vi "Upate Power.vi"(8 "error in":errorcluster, 11 "Refnum in":refnum<k21>) -> (0 "error out":errorcluster, 3 "Refnum out":refnum<k21>)   [LabVIEW 2015]
uses:
  <vilib>/DAQmx/write.llb/DAQmx Write (Digital 1D Bool NChan 1Samp 1Line).vi
  <vilib>/DAQmx/miscellaneous.llb/DAQmx Fill In Error Info.vi
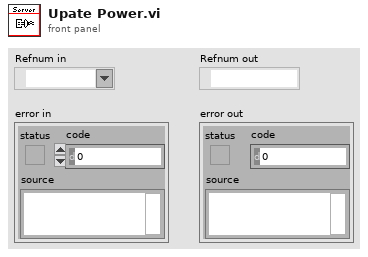
[diagram p1: front panel]
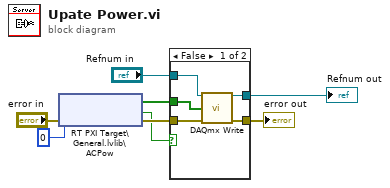
[diagram p0: block diagram]
diagram:
  n1 = shared-variable "RT PXI Target\\General.lvlib\\ACPow"(error in="error in", 0 ("ms timeout (0)")) -> (w8:bool[], error out=w6:errorcluster, w5:bool)
  n2 = case shown="False" w5 {
    tunnel: w6 -> [w12 w15]
    tunnel: w8 -> [w13 _]
    tunnel: [w11 w15] -> w2
    tunnel: "Refnum in" -> [w10 w14]
    tunnel: [w9 w14] -> w4
    frame False {
      n3 = call-poly <vilib>:"DAQmx Write.vi"("task/channels in"=w10, "data"=w13, "error in"=w12) -> ("task out"=w9:refnum<k21>, "error out"=w11:errorcluster)  [unwired: 10 in, 1 out]
    }
    frame True {
    }
  }
  "Refnum out" <- w4
  "error out" <- w2
